vi "String Date Time to Timestamp.vi"(8 "error in (no error)":errorcluster, 10 "Use milliseconds":bool=TRUE, 11 "String to Convert":string) -> (0 "error out":errorcluster, 3 "Timestamp Value":timestamp)   [LabVIEW 2023, in "HAF.lvlib"]
doc: "Converts the passed String value to Timestamp. The passed String must be in the format [Locale Date] [Locale Time] and milliseconds can be used. If not, a conversion or other error will be returned. Day and Month can be single digits, year must be 4 digits. Milliseconds portion can be specified in micro- or nano- etc, but will be truncated to milliseconds. Default is to use milliseconds."
uses:
  HAF.lvlib
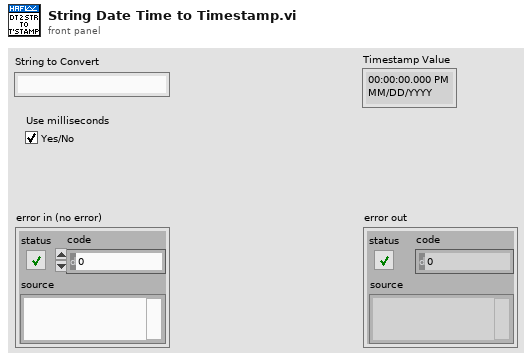
[diagram p1: front panel]
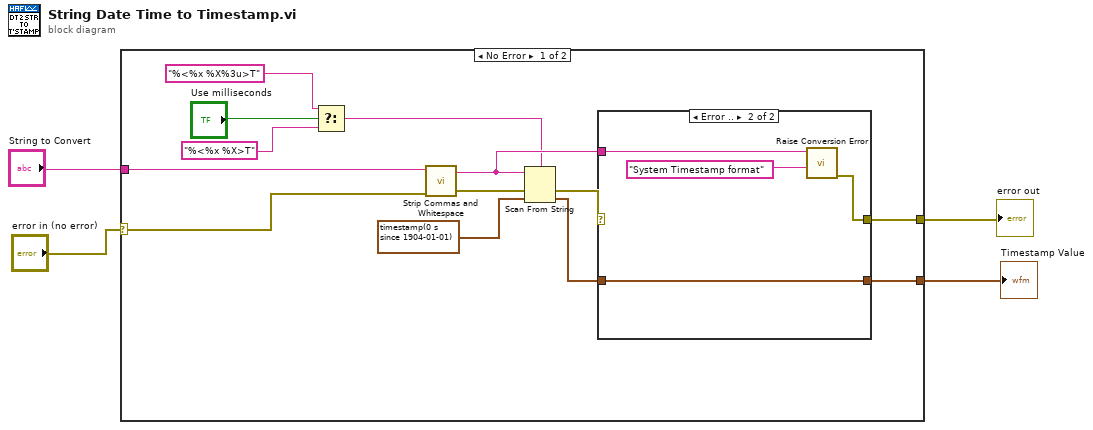
[diagram p0: block diagram]
diagram:
  n1 = case shown="No Error" "error in (no error)" {
    selector: "error in (no error)" -> [w16 w24]
    tunnel: "String to Convert" -> [w17 _]
    tunnel: [w13 w24] -> w2
    tunnel: [w12 _] -> w1
    frame No Error {
      n2 = Select(t="%<%x %X%3u>T" ("format string"), s="Use milliseconds", f="%<%x %X>T") -> (s? t:f=w7:string)
      n3 = call "Strip Commas and Whitespace.vi"("error in (no error)"=w16, "String to Strip"=w17) -> ("error out"=w15:errorcluster, "Clean String"=w11:string)  [unwired: 8 in]
      n4 = Scan From String(format string=w7, input string=w11, error in=w15, default 1=timestamp(0 s since 1904-01-01) ("default value 1")) -> (error out=w14:errorcluster, output 1=w5:timestamp)  [unwired: 1 in, 2 out]
      n5 = case shown="Error .." w14 {
        selector: w14 -> [w19 _]
        tunnel: w5 -> [w18 w20]
        tunnel: [w19 w21] -> w13
        tunnel: [w18 w20] -> w12
        tunnel: w11 -> [_ w23]
        frame No Error {
        }
        frame Error {
          n6 = call "Raise Conversion Error.vi"("Data Type Attempted"="System Timestamp format", "String in Error"=w23) -> ("error out"=w21:errorcluster)  [unwired: 9 in]
        }
      }
    }
    frame Error {
    }
  }
  "Timestamp Value" <- w1
  "error out" <- w2
